vi "Frequency Sweep.vi"(0 "Hardware.lvlib:Scope.lvclass":refnum<class "Scope.lvclass">, 1 "Hardware.lvlib:Function Generator.lvclass":refnum<class "Function Generator.lvclass">, 2 "Amplitude (1)":dbl=0.5, 3 "Number of Steps (25)":i32=25, 4 "Input Channel (1)":dbl=1.0, 5 "error in (no error)":errorcluster, 6 "Waveform Function (1: Sine)":u16(ring)=1 items=["DC", "Sine", "Square", "Triangle", "Ramp", "Pulse", "Noise", "Sinc", "Negative Ramp", "Exponential Rise", "Exponential Fall", "Cardiac"], 7 "Start Frequency (1000)":dbl=1000.0, 9 "Stop Frequency (50000)":dbl=50000.0) -> (14 "Hardware.lvlib:Scope.lvclass Out":refnum<class "Scope.lvclass">, 15 "Hardware.lvlib:Function Generator.lvclass Out":refnum<class "Function Generator.lvclass">, 16 "Freq Amp Array":dbl[][](array[numeric])=[[1000.0, 25750.0, 50500.0, 75250.0, 100000.0], [6.881057614454697, 0.7762788757172112, 3.877116497313211, 5.5398055148465115, 8.936592894514183]], 19 "error out":errorcluster)   [LabVIEW 2015, in "Frequency Measurement.lvlib" / "Frequency Measurement.lvclass"]
uses:
  Frequency Measurement.lvclass
  <userlib>/Common Components/Hardware/Scope/Scope.lvclass
  <userlib>/Common Components/Hardware/FGEN/Function Generator.lvclass
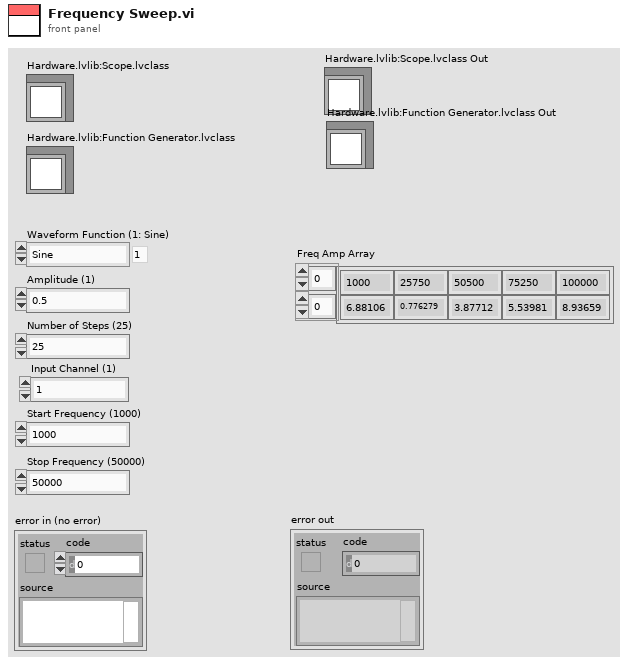
[diagram p1: front panel]
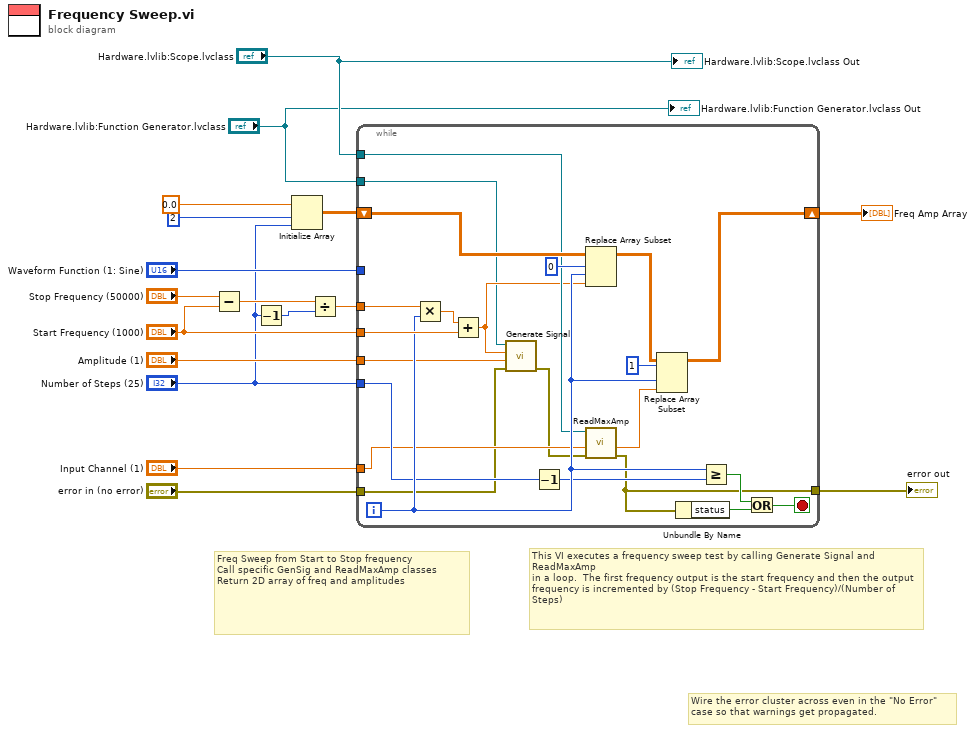
[diagram p0: block diagram]
diagram:
  # "This VI executes a frequency sweep test by calling Generate Signal and ReadMaxAmp\nin a loop.  The first frequency output is the start frequency and then the output frequency is incremented by (Stop Frequency - Start Frequency)/(Number of Steps)"
  # "Freq Sweep from Start to Stop frequency\nCall specific GenSig and ReadMaxAmp classes\nReturn 2D array of freq and amplitudes"
  # "Wire the error cluster across even in the \"No Error\"\ncase so that warnings get propagated."
  n1 = Subtract(x="Stop Frequency (50000)", y="Start Frequency (1000)") -> (x-y=w14:dbl)
  n2 = Decrement(x="Number of Steps (25)") -> (x-1=w6:i32)
  n3 = Initialize Array(0.0 ("element"), 2 ("dimension size"), "Number of Steps (25)") -> (w9:dbl[][])
  n4 = Divide(x=w14, y=w6) -> (x/y=w12:dbl)
  n5 = while {
    tunnel: "error in (no error)" -> [w19]
    tunnel: "Waveform Function (1: Sine)" -> [_]
    tunnel: [w26] -> w3
    tunnel: "Input Channel (1)" -> [w24]
    tunnel: "Hardware.lvlib:Function Generator.lvclass" -> [w21]
    tunnel: "Hardware.lvlib:Scope.lvclass" -> [w23]
    tunnel: "Start Frequency (1000)" -> [w39]
    tunnel: w12 -> [w38]
    tunnel: "Amplitude (1)" -> [w20]
    shift-right: [w33] -> w7
    shift-left: w9 -> [w37]
    tunnel: "Number of Steps (25)" -> [w28]
    i -> [w29]
    stop <- w31 stop-if-true
    n6 = Multiply(x=w38, y=w29) -> (x*y=w40:dbl)
    n7 = Add(x=w40, y=w39) -> (x+y=w22:dbl)
    n8 = call-dynamic "Generate Signal.vi"("error in (no error)"=w19, 9:w20, "Frequency (1000 Hz)"=w22, "Function Generator in"=w21) -> ("error out"=w18:errorcluster)  [unwired: 6 in, 1 out]
    n9 = Decrement(x=w28) -> (x-1=w27:i32)
    n10 = Replace Array Subset(array=w37, new element=w22, index (row)=0, index (col)=w29) -> (w35:dbl[][])
    n11 = call-dynamic "ReadMaxAmp.vi"("error in (no error)"=w18, "Channel"=w24, "Scope in"=w23) -> ("error out"=w26:errorcluster, "Amplitude"=w25:dbl)  [unwired: 7 out]
    n12 = Replace Array Subset(array=w35, new element=w25, index (row)=1, index (col)=w29) -> (w33:dbl[][])
    n13 = Unbundle By Name(w26) -> ("status"=w32:bool)
    n14 = Greater Or Equal?(x=w29, y=w27) -> (x >= y?=w30:bool)
    n15 = Or(x=w30, y=w32) -> (x .or. y?=w31:bool)
  }
  "error out" <- w3
  "Freq Amp Array" <- w7
  "Hardware.lvlib:Scope.lvclass Out" <- "Hardware.lvlib:Scope.lvclass"
  "Hardware.lvlib:Function Generator.lvclass Out" <- "Hardware.lvlib:Function Generator.lvclass"
